vi "Programa_robot_final_5.vi"() -> ()   [LabVIEW 2019]
uses:
  <vilib>/Instr/_visa.llb/VISA Configure Serial Port (Instr).vi
  Global_STOP.vi
  <vilib>/regexp/Match Regular Expression.xnode
panel:
  in  "Ruta hacia el fichero que contiene la imagen de la       superficie del ASIC  fotografiada por el microscopio":path=path "C:/Trabajo_Robot/Test Asic Javi_2021/Origen Socket SERVO_PCB_BUENO_v5 (muchos asics)/capturaQR.jpg"
  in  "stop 6":bool
  in  "Abrir socket 2":bool
  in  "Cerrar socket 2":bool
  in  "Interruptor Error 2":bool
  in  "stop 5":bool
  out "Datos_QR 3":string
  out "Existe foto anterior?":bool
  in  "STOP TEST 3":bool
  in  "stop socket 4":bool
  in  "stop 4":bool
  in  "stop 3":bool
  in  "stop 2":bool
  in  "stop socket 3":bool
  in  "Interruptor Error":bool
  in  "Cerrar socket":bool
  in  "Abrir socket":bool
  out "Error_QR":bool
  out "return count":u32
  out "lectura puerto serie":u32
  out "dato escrito puerto serie":string
  out "OK, Fault 2":bool
  out "error out":errorcluster {"code" format="%f"}
  in  "STOP TEST 2":bool
  out "Datos_QR 2":string
  out "NUMERO ASICS TESTEADOS":i32
  out ".not. x?":bool
  in  "Config File":path=path "C:/Trabajo_Robot/Test Asic Javi_2021/Origen Socket SERVO_PCB_BUENO_v5 (muchos asics)/CONFIG/configuracion_robot_CTAV2022A.test"
  in  "SELECCION DE TEST":string(combo)
  in  "?":bool
  out "Boolean":bool
  in  "stop socket 2":bool
  out "Bytes at port 3":u32=1
  in  "IN y":string(combo)="00"
  in  "IN x":string(combo)="00"
  in  "NOK y":string(combo)="00"
  in  "NOK x":string(combo)="00"
  in  "OK y":string(combo)="00"
  in  "OK x":string(combo)="00"
  in  "Operator's name":string(combo)="Juan Rodríguez"
  in  "?":bool
  in  "Fichero de registro":path=path "C:/Trabajo_Robot/Pruebas/Pruebas.txt"
  in  "Path Out Report":path=path "C:/Trabajo_Robot/desde Marzo 2023/Pruebas_PC_APD/RESULT_TEST_C_LABP0"
  in  "stop socket":bool
  out "Bytes at port 1":u32
  out "Iteraciones":i32
  out "Lectura buffer":string="1"
  in  "Delay (ms)":dbl=1.0 min=1.0 max=9.0 step=1.0
  out "Bytes at port 2":u32=1
  in  "Interruptor":bool=TRUE
  in  "stop":bool
  # "SI SE PRESIONA EL BOTON STOP PARA DETENER EL TEST,\nHAY QUE APAGAR Y VOLVER A ENCENDER EL ARDUINO"
  # "x: columna en cada bandeja \ny: fila en cada bandeja"
  # "Funcionamiento: en la primera iteración, el efector se desplaza desde el origen hasta la celda\nintroducida, hace una pausa, va a la posición del socket (0,0), hace otra pausa, va a la celda\nde salida y vuelve al origen. En las iteraciones siguientes hará lo mismo pero recorriendo las\nceldas de la bandeja sucesivamente. Que el desplazamiento se produzca hacia una celda de\nla bandeja OK o de la bandeja NOK depende de la salidad del programa de test de Asics."
types:
  T1 = enum16{"open", "replace", "create", "open or create", "replace or create", "replace or create with confirmation"}
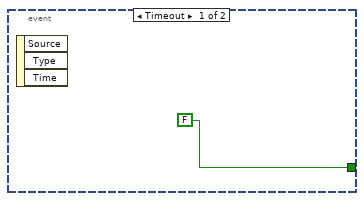
[diagram p2: hidden frame]
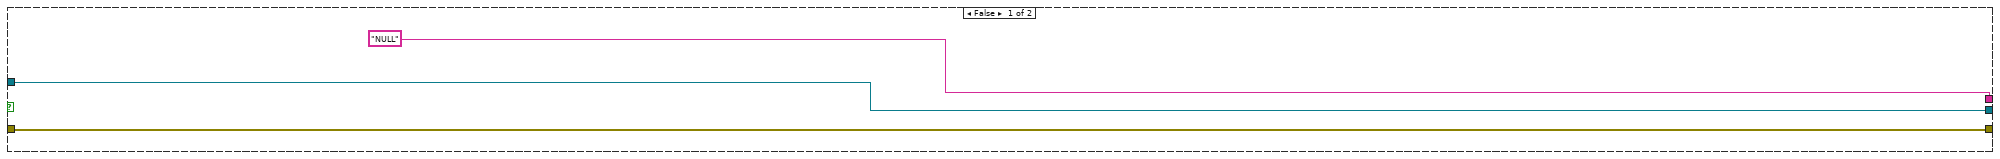
[diagram p5: hidden frame]
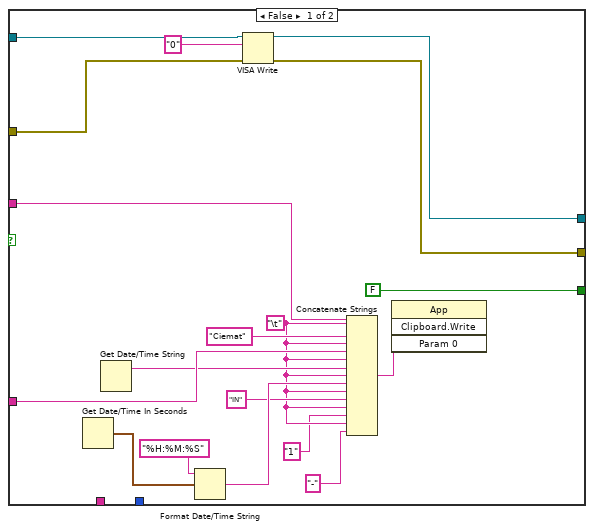
[diagram p8: hidden frame]
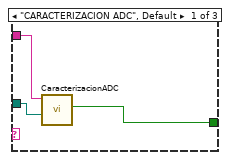
[diagram p9: hidden frame]
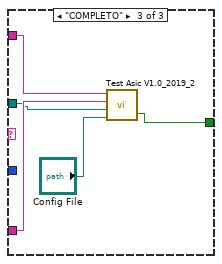
[diagram p10: hidden frame]
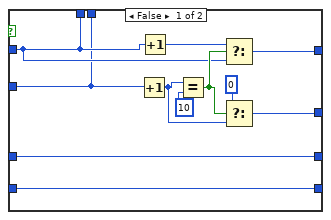
[diagram p12: hidden frame]
diagram:
  n1 = control-ref of="stop socket"() -> (w1:refnum<vi>)
  n2 = control-ref of="Cerrar socket"() -> (w9:refnum<vi>)
  n3 = control-ref of="STOP TEST 2"() -> (w12:refnum<vi>)
  n4 = control-ref of="Abrir socket"() -> (w7:refnum<vi>)
  n5 = control-ref of="stop"() -> (w8:refnum<vi>)
  n6 = control-ref of="Interruptor Error"() -> (w10:refnum<vi>)
  n7 = property class="Bool (strict)"(reference=w12, "Visible"=FALSE) -> ()  [unwired: 1 in, 2 out]
  n8 = property class="Bool (strict)"(reference=w7, "Visible"=FALSE) -> ()  [unwired: 1 in, 2 out]
  n9 = property class="Bool (strict)"(reference=w10, "Visible"=FALSE) -> ()  [unwired: 1 in, 2 out]
  n10 = property class="Bool (strict)"(reference=w9, "Visible"=FALSE) -> ()  [unwired: 1 in, 2 out]
  n11 = property on="Boolean" class="Bool (strict)"("Visible"=FALSE) -> ()  [unwired: 2 in, 2 out]
  n12 = property class="Bool"(reference=w1, "Visible"=FALSE) -> ()  [unwired: 1 in, 2 out]
  n13 = property class="Bool"(reference=w8, "Visible"=FALSE) -> ()  [unwired: 1 in, 2 out]
  n14 = flat-sequence {
    tunnel: [w54] -> w18
    tunnel: ["Fichero de registro"] -> w17
    tunnel: ["SELECCION DE TEST"] -> w16
    tunnel: ["NOK y"] -> w33
    tunnel: ["NOK x"] -> w32
    tunnel: ["OK y"] -> w31
    tunnel: ["OK x"] -> w30
    tunnel: ["IN y"] -> w29
    tunnel: ["IN x"] -> w28
    tunnel: [w57] -> w27
    tunnel: [w58] -> w26
    tunnel: ["IN y"] -> w25
    tunnel: ["IN x"] -> w24
    tunnel: w17 -> [w56]
    frame #0 {
      n15 = while {
        stop <- "?" stop-if-true
        n16 = Not(x="?") -> (.not. x?=w50:bool)
        "Boolean" <- w50
        n17 = property on="Boolean" class="Bool (strict)"("Blinking"=w50) -> ()  [unwired: 2 in, 2 out]
      }
      n18 = global write "Global_STOP.vi" "stop"(FALSE ("stop")) -> ()
    }
    frame #1 {
      n19 = Not(x="?") -> (.not. x?=w54:bool)
      ".not. x?" <- w54
    }
    frame #2 {
      n20 = Open/Create/Replace File(file path (use dialog)=w56, operation (0:open)=T1."open", access (0:read/write)=enum16{"read/write", "read-only", "write-only"}."write-only") -> (refnum out=w69:refnum<file>, error out=w71:errorcluster)  [unwired: 3 in, 1 out]
      n21 = Set File Position(refnum=w69, from (0:start)=enum16{"start", "end", "current"}."end", error in=w71) -> (refnum out=w70:refnum<file>, error out=w72:errorcluster)  [unwired: 1 in]
      n22 = Write to Text File(file (use dialog)=w70, text="\r\n", error in=w72) -> (refnum out=w58:refnum<file>, error out=w57:errorcluster)  [unwired: 1 in, 1 out]
    }
  }
  n23 = Decimal String To Number(string=w25) -> (number=w23:i32)  [unwired: 2 in, 1 out]
  n24 = Decimal String To Number(string=w24) -> (number=w20:i32)  [unwired: 2 in, 1 out]
  n25 = Multiply(x=10, y=w23) -> (x*y=w21:i32)
  n26 = Decimal String To Number(string=w31) -> (number=w35:i32)  [unwired: 2 in, 1 out]
  n27 = Decimal String To Number(string=w30) -> (number=w34:i32)  [unwired: 2 in, 1 out]
  n28 = Decimal String To Number(string=w33) -> (number=w37:i32)  [unwired: 2 in, 1 out]
  n29 = Decimal String To Number(string=w32) -> (number=w36:i32)  [unwired: 2 in, 1 out]
  n30 = call-poly "VISA Configure Serial Port"("VISA resource name"=refnum<visa-resource-name> "COM9", "baud rate (9600)"=u32 9600, "data bits (8)"=u16 8) -> ("VISA resource name out"=w41:refnum<visa-resource-name>, "error out"=w44:errorcluster)  [unwired: 11 in]
  n31 = Add(x=w21, y=w20) -> (x+y=w19:i32)
  n32 = while {
    shift-right: [w82] -> w42
    shift-left: w44 -> [w123]
    tunnel: w41 -> [w121]
    tunnel: [w84] -> w43
    tunnel: w26 -> [w114]
    tunnel: [w113] -> w40
    tunnel: w27 -> [w112]
    tunnel: [w111] -> w39
    tunnel: w28 -> [w109]
    tunnel: w29 -> [w108]
    tunnel: w30 -> [w107]
    tunnel: w31 -> [w106]
    tunnel: w32 -> [w105]
    tunnel: w33 -> [w104]
    shift-right: [w97] -> _
    shift-left: w37 -> [w103]
    shift-right: [w99] -> _
    shift-left: w36 -> [w102]
    shift-right: [w96] -> _
    shift-left: w35 -> [w101]
    shift-right: [w98] -> _
    shift-left: w34 -> [w100]
    tunnel: w19 -> [w95]
    tunnel: w18 -> [w87]
    tunnel: w16 -> [w86]
    tunnel: [w80] -> w14
    i -> [w85]
    stop <- w80 stop-if-true
    n33 = flat-sequence {
      tunnel: w123 -> [w176]
      tunnel: w121 -> [w165]
      tunnel: [w167] -> w120
      tunnel: [w166] -> w119
      tunnel: w109 -> [w146]
      tunnel: w108 -> [w145]
      tunnel: w107 -> [w144]
      tunnel: w106 -> [w143]
      tunnel: w105 -> [w142]
      tunnel: w104 -> [w141]
      tunnel: w120 -> [w913]
      tunnel: w119 -> [w912]
      tunnel: [w911] -> w94
      tunnel: [w910] -> w92
      tunnel: [w909] -> _
      tunnel: w94 -> [w929]
      tunnel: [w927] -> w93
      tunnel: w92 -> [w928]
      tunnel: [w926] -> w91
      tunnel: w93 -> [w949]
      tunnel: w91 -> [w948]
      tunnel: w85 -> [w950]
      tunnel: [w946] -> w90
      tunnel: [w945] -> w89
      tunnel: [w944] -> w88
      tunnel: w85 -> [w1059]
      tunnel: [w1061] -> w117
      tunnel: [w1060] -> w116
      tunnel: [w1057] -> w110
      tunnel: w90 -> [w1056]
      tunnel: w89 -> [w1055]
      tunnel: w88 -> [w1054]
      tunnel: w87 -> [w1049]
      tunnel: w86 -> [w1052]
      tunnel: w85 -> [w1051]
      tunnel: [w1122] -> w115
      tunnel: [w1124] -> w118
      tunnel: w117 -> [w1123]
      tunnel: w116 -> [w1121]
      tunnel: w114 -> [w1128]
      tunnel: [w1127] -> w113
      tunnel: w112 -> [w1126]
      tunnel: [w1125] -> w111
      tunnel: w85 -> [w1118]
      tunnel: w110 -> [w1117]
      tunnel: w103 -> [w1113]
      tunnel: w102 -> [w1116]
      tunnel: w101 -> [w1115]
      tunnel: w100 -> [w1114]
      tunnel: [w1112] -> w97
      tunnel: [w1111] -> w99
      tunnel: [w1110] -> w96
      tunnel: [w1109] -> w98
      tunnel: w95 -> [w1108]
      tunnel: w85 -> [w1107]
      tunnel: [w1106] -> _
      frame #0 {
        n34 = for {
          N: 2 -> [_]
          shift-right: [w788] -> _
          shift-left: w146 -> [w793]
          shift-right: [w791] -> w162
          shift-left: w165 -> [w792]
          shift-right: [w789] -> w161
          shift-left: w176 -> [w790]
          n35 = xnode "Match Regular Expression"("input string"=w793, "regular expression"="-?\\d") -> ("whole match"=w787:string, "after match"=w788:string)  [unwired: 4 in, 3 out]
          n36 = VISA Write(VISA resource name=w792, write buffer=w787, error in (no error)=w790) -> (VISA resource name out=w791:refnum<visa-resource-name>, error out=w789:errorcluster)  [unwired: 1 out]
        }
        n37 = for {
          N: 2 -> [_]
          shift-right: [w666] -> _
          shift-left: w145 -> [w671]
          shift-right: [w669] -> w156
          shift-left: w162 -> [w670]
          shift-right: [w667] -> w155
          shift-left: w161 -> [w668]
          n38 = xnode "Match Regular Expression"("input string"=w671, "regular expression"="-?\\d") -> ("whole match"=w665:string, "after match"=w666:string)  [unwired: 4 in, 3 out]
          n39 = VISA Write(VISA resource name=w670, write buffer=w665, error in (no error)=w668) -> (VISA resource name out=w669:refnum<visa-resource-name>, error out=w667:errorcluster)  [unwired: 1 out]
        }
        n40 = for {
          N: 2 -> [_]
          shift-right: [w544] -> _
          shift-left: w144 -> [w549]
          shift-right: [w547] -> w158
          shift-left: w156 -> [w548]
          shift-right: [w545] -> w157
          shift-left: w155 -> [w546]
          n41 = xnode "Match Regular Expression"("input string"=w549, "regular expression"="-?\\d") -> ("whole match"=w543:string, "after match"=w544:string)  [unwired: 4 in, 3 out]
          n42 = VISA Write(VISA resource name=w548, write buffer=w543, error in (no error)=w546) -> (VISA resource name out=w547:refnum<visa-resource-name>, error out=w545:errorcluster)  [unwired: 1 out]
        }
        n43 = for {
          N: 2 -> [_]
          shift-right: [w422] -> _
          shift-left: w143 -> [w427]
          shift-right: [w425] -> w150
          shift-left: w158 -> [w426]
          shift-right: [w423] -> w149
          shift-left: w157 -> [w424]
          n44 = xnode "Match Regular Expression"("input string"=w427, "regular expression"="-?\\d") -> ("whole match"=w421:string, "after match"=w422:string)  [unwired: 4 in, 3 out]
          n45 = VISA Write(VISA resource name=w426, write buffer=w421, error in (no error)=w424) -> (VISA resource name out=w425:refnum<visa-resource-name>, error out=w423:errorcluster)  [unwired: 1 out]
        }
        n46 = for {
          N: 2 -> [_]
          shift-right: [w300] -> _
          shift-left: w142 -> [w305]
          shift-right: [w303] -> w152
          shift-left: w150 -> [w304]
          shift-right: [w301] -> w151
          shift-left: w149 -> [w302]
          n47 = xnode "Match Regular Expression"("input string"=w305, "regular expression"="-?\\d") -> ("whole match"=w299:string, "after match"=w300:string)  [unwired: 4 in, 3 out]
          n48 = VISA Write(VISA resource name=w304, write buffer=w299, error in (no error)=w302) -> (VISA resource name out=w303:refnum<visa-resource-name>, error out=w301:errorcluster)  [unwired: 1 out]
        }
        n49 = for {
          N: 2 -> [_]
          shift-right: [w178] -> _
          shift-left: w141 -> [w183]
          shift-right: [w181] -> w148
          shift-left: w152 -> [w182]
          shift-right: [w179] -> w147
          shift-left: w151 -> [w180]
          n50 = xnode "Match Regular Expression"("input string"=w183, "regular expression"="-?\\d") -> ("whole match"=w177:string, "after match"=w178:string)  [unwired: 4 in, 3 out]
          n51 = VISA Write(VISA resource name=w182, write buffer=w177, error in (no error)=w180) -> (VISA resource name out=w181:refnum<visa-resource-name>, error out=w179:errorcluster)  [unwired: 1 out]
        }
        n52 = Number To Decimal String(number="Delay (ms)") -> (decimal integer string=w170:string)  [unwired: 1 in]
        n53 = VISA Write(VISA resource name=w148, write buffer=w170, error in (no error)=w147) -> (VISA resource name out=w172:refnum<visa-resource-name>, error out=w171:errorcluster)  [unwired: 1 out]
        n54 = Select(t="1" ("write buffer"), s="Interruptor", f="0" ("write buffer")) -> (s? t:f=w168:string)
        n55 = VISA Write(VISA resource name=w172, write buffer=w168, error in (no error)=w171) -> (VISA resource name out=w167:refnum<visa-resource-name>, error out=w166:errorcluster)  [unwired: 1 out]
      }
      frame #1 {
        n56 = while {
          shift-right: [w919] -> w910
          shift-left: w912 -> [w924]
          tunnel: ["stop socket"] -> _
          shift-right: [w920] -> w911
          shift-left: w913 -> [w925]
          tunnel: ["stop socket"] -> w909
          stop <- w914 stop-if-true
          n57 = property class="Instr"(reference=w925, error in=w924) -> (reference out=w923:refnum<visa-resource-name>, error out=w922:errorcluster, "Bytes at Port"=w921:u32)
          "Bytes at port 1" <- w921
          n58 = VISA Read(VISA resource name=w923, byte count=w921, error in (no error)=w922) -> (VISA resource name out=w920:refnum<visa-resource-name>, read buffer=w918:string, error out=w919:errorcluster)  [unwired: 1 out]
          n59 = Equal?(x="2", y=w918) -> (x = y?=w916:bool)
          n60 = Or(x=w916, y="stop socket") -> (x .or. y?=w914:bool)
        }
      }
      frame #2 {
        n61 = while {
          shift-right: [w935] -> w926
          shift-left: w928 -> [w940]
          tunnel: ["stop socket 2"] -> _
          shift-right: [w936] -> w927
          shift-left: w929 -> [w941]
          tunnel: ["stop socket 2"] -> _
          stop <- w930 stop-if-true
          n62 = property class="Instr"(reference=w941, error in=w940) -> (reference out=w939:refnum<visa-resource-name>, error out=w938:errorcluster, "Bytes at Port"=w937:u32)
          "Bytes at port 3" <- w937
          n63 = VISA Read(VISA resource name=w939, byte count=w937, error in (no error)=w938) -> (VISA resource name out=w936:refnum<visa-resource-name>, read buffer=w934:string, error out=w935:errorcluster)  [unwired: 1 out]
          n64 = Equal?(x="3", y=w934) -> (x = y?=w932:bool)
          n65 = Or(x=w932, y="stop socket 2") -> (x .or. y?=w930:bool)
        }
      }
      frame #3 {
        # "Este bloque realiza la captura y lectura del QR"
        n66 = Greater?(x=w950, y=-1) -> (0:w947:bool)
        n67 = case shown="True" w947 {
          tunnel: [w954 w956] -> w944
          tunnel: w949 -> [w954 w958]
          tunnel: [w953 w957] -> w946
          tunnel: w948 -> [w953 w959]
          tunnel: ["NULL" ("Datos_QR") w955] -> w945
          frame False {
          }
          frame True {
            n68 = while {
              tunnel: [w965] -> w955
              tunnel: w958 -> [w976]
              tunnel: [w972] -> w956
              tunnel: [w971] -> w957
              tunnel: w959 -> [w966]
              stop <- w961 stop-if-true
              n69 = flat-sequence {
                tunnel: [w980] -> w967
                tunnel: w966 -> [w978]
                tunnel: [w992] -> w965
                tunnel: [w990] -> w962
                tunnel: w967 -> [w989]
                tunnel: [w989] -> w964
                frame #0 {
                  # "Éste bloque borra el fichero de imagen\ndel Asic anterior."
                  n70 = call <vilib>:"Check if File or Folder Exists.vi"("error in (no error)"=w978, "path"="Ruta hacia el fichero que contiene la imagen de la       superficie del ASIC  fotografiada por el microscopio") -> ("error out"=w979:errorcluster, "file or folder exists?"=w982:bool, "dup path"=w981:path)  [unwired: 7 in]
                  "Existe foto anterior?" <- w982
                  n71 = case shown="True" w982 {
                    tunnel: w981 -> [w984 w988]
                    tunnel: [w984 w987] -> _
                    tunnel: [w983 w986] -> w980
                    tunnel: w979 -> [w983 w985]
                    frame False {
                    }
                    frame True {
                      n72 = Delete(path (use dialog)=w988, error in=w985) -> (deleted path=w987:path, error out=w986:errorcluster)  [unwired: 3 in, 1 out]
                    }
                  }
                }
                frame #1 {
                  # "Éste bloque realiza la captura de imagen\ndel QR del asic para leer el código."
                  n73 = for {
                    N: 5 -> [_]
                    tunnel: [w997] -> w992
                    tunnel: [w995] -> w990
                    stop <- w993 stop-if-true
                    n74 = call "CapturaImagenyQR_subVI.vi"() -> ("Datos_QR"=w997:string)  [unwired: 11 in]
                    "Datos_QR 3" <- w997
                    n75 = Equal?(x=w997, y="" ("Datos_QR")) -> (x = y?=w996:bool)
                    n76 = global read "Global_STOP.vi" "stop"() -> (w994:bool)
                    n77 = Not(x=w996) -> (.not. x?=w995:bool)
                    n78 = Compound Arithmetic op=OR(w995, w994) -> (w993:bool)
                  }
                }
              }
              n79 = Select(t="1" ("write buffer"), s=w962, f="0" ("write buffer")) -> (s? t:f=w973:string)
              n80 = Not(x=w962) -> (.not. x?=→"Error_QR":bool)
              n81 = VISA Write(VISA resource name=w976, write buffer=w973, error in (no error)=w964) -> (VISA resource name out=w970:refnum<visa-resource-name>, error out=w969:errorcluster)  [unwired: 1 out]
              n82 = global read "Global_STOP.vi" "stop"() -> (w963:bool)
              n83 = case shown="False" w962 {
                tunnel: w970 -> [w1010 w1045]
                tunnel: w969 -> [w1009 w1044]
                tunnel: [w1008 w1045] -> w972
                tunnel: [w1007 w1044] -> w971
                frame False {
                  n84 = flat-sequence {
                    tunnel: w1010 -> [w1014]
                    tunnel: [w1013] -> w1006
                    tunnel: [w1012] -> w1004
                    tunnel: w1009 -> [w1011]
                    tunnel: w1006 -> [w1025]
                    tunnel: [w1025] -> w1005
                    tunnel: w1004 -> [w1024]
                    tunnel: [w1024] -> w1003
                    tunnel: w1005 -> [w1029]
                    tunnel: w1003 -> [w1028]
                    tunnel: [w1027] -> w1002
                    tunnel: [w1026] -> w1000
                    tunnel: w1002 -> [w1040]
                    tunnel: [w1040] -> w1001
                    tunnel: w1000 -> [w1039]
                    tunnel: [w1039] -> w999
                    tunnel: [w1041] -> w1007
                    tunnel: [w1042] -> w1008
                    tunnel: w1001 -> [w1042]
                    tunnel: w999 -> [w1041]
                    frame #0 {
                      n85 = while {
                        tunnel: w1014 -> [w1022]
                        tunnel: [w1017] -> w1013
                        tunnel: [w1016] -> w1012
                        tunnel: w1011 -> [w1015]
                        stop <- "Abrir socket" stop-if-true
                        n86 = Select(t="2" ("write buffer"), s="Abrir socket", f="0" ("write buffer")) -> (s? t:f=w1019:string)
                        n87 = VISA Write(VISA resource name=w1022, write buffer=w1019, error in (no error)=w1015) -> (VISA resource name out=w1017:refnum<visa-resource-name>, error out=w1016:errorcluster)  [unwired: 1 out]
                      }
                    }
                    frame #1 {
                      n88 = Wait (ms)(milliseconds to wait=u32 1000) -> ()  [unwired: 1 out]
                    }
                    frame #2 {
                      n89 = while {
                        tunnel: w1029 -> [w1033]
                        tunnel: w1028 -> [w1032]
                        tunnel: [w1031] -> w1027
                        tunnel: [w1030] -> w1026
                        stop <- "Cerrar socket" stop-if-true
                        n90 = Select(t="3" ("write buffer"), s="Cerrar socket", f="0" ("write buffer")) -> (s? t:f=w1035:string)
                        n91 = VISA Write(VISA resource name=w1033, write buffer=w1035, error in (no error)=w1032) -> (VISA resource name out=w1031:refnum<visa-resource-name>, error out=w1030:errorcluster)  [unwired: 1 out]
                      }
                    }
                    frame #3 {
                      n92 = Wait (ms)(milliseconds to wait=u32 1000) -> ()  [unwired: 1 out]
                    }
                    frame #4 {
                      n93 = while {
                        stop <- "Interruptor Error" stop-if-true
                      }
                    }
                  }
                }
                frame True {
                }
              }
              n94 = Or(x=w962, y=w963) -> (x .or. y?=w961:bool)
            }
            n95 = Wait (ms)(milliseconds to wait=u32 10000) -> ()  [unwired: 1 out]
          }
        }
        n96 = control-ref of="STOP TEST 2"() -> (w943:refnum<vi>)
        n97 = property class="Bool (strict)"(reference=w943, "Visible"=TRUE) -> ()  [unwired: 1 in, 2 out]
      }
      frame #4 {
        n98 = global read "Global_STOP.vi" "stop"() -> (w1048:bool)
        n99 = Greater?(x=w1059, y=-1) -> (0:w1050:bool)
        n100 = Not(x=w1048) -> (.not. x?=w1047:bool)
        n101 = Compound Arithmetic op=AND(w1050, w1049, w1047) -> (w1046:bool)
        n102 = case shown="True" w1046 {
          tunnel: w1054 -> [w1077 w1084]
          tunnel: w1056 -> [w1076 w1083]
          tunnel: [w1075 w1082] -> w1061
          tunnel: [w1074 w1081] -> w1060
          tunnel: w1055 -> [w1070 w1091]
          tunnel: [FALSE ("Boolean") w1089] -> w1057
          tunnel: "Operator's name" -> [w1068 w1088]
          tunnel: w1052 -> [_ w1087]
          tunnel: w1051 -> [_ w1086]
          frame False {
            w1064 = "\t"
            n103 = Get Date/Time In Seconds() -> (seconds since 1Jan1904=w1072:timestamp)
            n104 = Get Date/Time String() -> (date string=w1067:string)  [unwired: 3 in, 1 out]
            n105 = Format Date/Time String(time format string (%c)="%H:%M:%S", seconds (now)=w1072) -> (date/time string=w1066:string)  [unwired: 1 in]
            n106 = VISA Write(VISA resource name=w1077, write buffer="0", error in (no error)=w1076) -> (VISA resource name out=w1075:refnum<visa-resource-name>, error out=w1074:errorcluster)  [unwired: 1 out]
            n107 = Concatenate Strings(w1070, w1064, "Ciemat", w1064, w1068, w1064, w1067, w1064, w1066, w1064, "IN", w1064, "1", w1064, "-") -> (w1073:string)
            n108 = invoke class="App" method="Clipboard.Write"("Param 0"=w1073) -> ()  [unwired: 3 in, 4 out]
          }
          frame True {
            # "Test de Asics"
            n109 = case shown="\"SUMAS 3 CANALES\"" w1087 {
              tunnel: w1091 -> [w1096 w1098 w1105]
              tunnel: "Path Out Report" -> [w1095 w1100 w1103]
              tunnel: [w1094 w1099 w1101] -> w1089
              tunnel: w1088 -> [_ _ w1104]
              tunnel: w1086 -> [_ w1097 _]
              frame "CARACTERIZACION ADC", Default {
                n110 = call "CaracterizacionADC.vi"("QR code"=w1096, "Path Out Report"=w1095) -> ("OK/NOK"=w1094:bool)  [unwired: 7 in]
              }
              frame "SUMAS 3 CANALES" {
                n111 = call "Test_Sumadores_Javi.vi"("QR"=w1098, "Path"=w1100, "NUMERO DE PASADA DE TEST"=w1097) -> ("Boolean"=w1099:bool)  [unwired: 8 in]
                "NUMERO ASICS TESTEADOS" <- w1097
              }
              frame "COMPLETO" {
                n112 = call "Test Asic V1.0_2019_2.vi"("Config File"="Config File", "Path Out Report"=w1103, "Operator's Name"=w1104, "ASIC'S Number"=w1105) -> ("OK, Fault 2"=w1101:bool)  [unwired: 1 in]
              }
            }
            "OK, Fault 2" <- w1089
            n113 = Select(t="1" ("write buffer"), s=w1089, f="0" ("write buffer")) -> (s? t:f=w1085:string)
            "dato escrito puerto serie" <- w1085
            n114 = VISA Write(VISA resource name=w1084, write buffer=w1085, error in (no error)=w1083) -> (VISA resource name out=w1082:refnum<visa-resource-name>, return count=→"return count":u32, error out=w1081:errorcluster)
          }
        }
      }
      frame #5 {
        n115 = Greater?(x=w1118, y=-1) -> (0:w1119:bool)
        n116 = case shown="True" w1119 {
          tunnel: w1128 -> [w1134 w1167]
          tunnel: [w1134 w1166] -> w1127
          tunnel: w1126 -> [w1133 w1165]
          tunnel: [w1133 w1164] -> w1125
          tunnel: [w1136 w1163] -> w1124
          tunnel: w1123 -> [w1136 w1163]
          tunnel: [w1135 w1162] -> w1122
          tunnel: w1121 -> [w1135 w1162]
          tunnel: w1117 -> [_ w1160]
          tunnel: w1113 -> [w1132 w1159]
          tunnel: w1116 -> [w1131 w1158]
          tunnel: w1115 -> [w1130 w1157]
          tunnel: w1114 -> [w1129 w1156]
          tunnel: [w1132 w1155] -> w1112
          tunnel: [w1131 w1154] -> w1111
          tunnel: [w1130 w1153] -> w1110
          tunnel: [w1129 w1152] -> w1109
          frame False {
          }
          frame True {
            w1139 = "\t"
            # "Registro de datos en fichero"
            n117 = invoke class="App" method="Clipboard.Read"() -> ("Read Clipbrd"=w1161:string)  [unwired: 3 in, 2 out]
            n118 = case shown="True" w1160 {
              tunnel: w1159 -> [w1170 w1183]
              tunnel: w1158 -> [w1169 w1182]
              tunnel: w1157 -> [w1172 w1180]
              tunnel: w1156 -> [w1171 w1181]
              tunnel: [w1174 w1183] -> w1155
              tunnel: [w1173 w1182] -> w1154
              tunnel: [w1172 w1185] -> w1153
              tunnel: [w1171 w1184] -> w1152
              tunnel: [w1170 w1180] -> w1151
              tunnel: [w1169 w1181] -> w1150
              frame False {
                n119 = Increment(x=w1169) -> (x+1=w1178:i32)
                n120 = Increment(x=w1170) -> (x+1=w1175:i32)
                n121 = Equal?(x=w1178, y=10) -> (x = y?=w1176:bool)
                n122 = Select(t=w1175, s=w1176, f=w1170) -> (s? t:f=w1174:i32)
                n123 = Select(t=0, s=w1176, f=w1178) -> (s? t:f=w1173:i32)
              }
              frame True {
                n124 = Increment(x=w1181) -> (x+1=w1189:i32)
                n125 = Increment(x=w1180) -> (x+1=w1186:i32)
                n126 = Equal?(x=w1189, y=10) -> (x = y?=w1187:bool)
                n127 = Select(t=w1186, s=w1187, f=w1180) -> (s? t:f=w1185:i32)
                n128 = Select(t=0, s=w1187, f=w1189) -> (s? t:f=w1184:i32)
              }
            }
            n129 = Write to Text File(file (use dialog)=w1167, text=w1161, error in=w1165) -> (refnum out=w1148:refnum<file>, error out=w1149:errorcluster)  [unwired: 1 in, 1 out]
            n130 = Number To Decimal String(number=w1151) -> (decimal integer string=w1138:string)  [unwired: 1 in]
            n131 = Number To Decimal String(number=w1150) -> (decimal integer string=w1137:string)  [unwired: 1 in]
            n132 = Write to Text File(file (use dialog)=w1148, text=w1139, error in=w1149) -> (refnum out=w1146:refnum<file>, error out=w1147:errorcluster)  [unwired: 1 in, 1 out]
            n133 = Write to Text File(file (use dialog)=w1146, text=w1138, error in=w1147) -> (refnum out=w1143:refnum<file>, error out=w1142:errorcluster)  [unwired: 1 in, 1 out]
            n134 = Write to Text File(file (use dialog)=w1143, text=w1139, error in=w1142) -> (refnum out=w1141:refnum<file>, error out=w1140:errorcluster)  [unwired: 1 in, 1 out]
            n135 = Write to Text File(file (use dialog)=w1141, text=w1137, error in=w1140) -> (refnum out=w1145:refnum<file>, error out=w1144:errorcluster)  [unwired: 1 in, 1 out]
            n136 = Write to Text File(file (use dialog)=w1145, text="\r\n", error in=w1144) -> (refnum out=w1166:refnum<file>, error out=w1164:errorcluster)  [unwired: 1 in, 1 out]
          }
        }
        n137 = Add(x=w1108, y=w1107) -> (x+y=w1106:i32)
      }
    }
    n138 = while {
      shift-right: [w1198] -> w76
      shift-left: w115 -> [w1204]
      tunnel: ["stop"] -> _
      shift-right: [w1199] -> w84
      shift-left: w118 -> [w1205]
      tunnel: [w1194] -> w122
      stop <- w1192 stop-if-true
      # "1"
      # "Mientras se ejecuta este bucle (la espera a que\nArduino termine una iteración), cambiamos los\ndatos de los controladores."
      n139 = property class="Instr"(reference=w1205, error in=w1204) -> (reference out=w1202:refnum<visa-resource-name>, error out=w1201:errorcluster, "Bytes at Port"=w1200:u32)
      "Bytes at port 2" <- w1200
      n140 = VISA Read(VISA resource name=w1202, byte count=w1200, error in (no error)=w1201) -> (VISA resource name out=w1199:refnum<visa-resource-name>, read buffer=w1194:string, return count=w1197:u32, error out=w1198:errorcluster)
      "lectura puerto serie" <- w1197
      n141 = Greater Or Equal?(x=w1197, y=u32 1) -> (x >= y?=w1195:bool)
      n142 = global read "Global_STOP.vi" "stop"() -> (w1191:bool)
      n143 = Or(x=w1195, y="stop") -> (x .or. y?=w1193:bool)
      n144 = Compound Arithmetic op=OR(w1193, w1191) -> (w1192:bool)
    }
    "Lectura buffer" <- w122
    n145 = flat-sequence {
      tunnel: w76 -> [w125]
      tunnel: [w125] -> w75
      tunnel: [w124] -> w73
      frame #0 {
        n146 = global read "Global_STOP.vi" "stop"() -> (w124:bool)
      }
    }
    n147 = case shown="False" w73 {
      selector: w73 -> [_ w135]
      tunnel: [w129 _] -> w81
      tunnel: [w126 w135] -> w77
      tunnel: w75 -> [w127 w134]
      tunnel: [w127 w134] -> w74
      frame False {
        n148 = for {
          N: 3 -> [_]
          tunnel: [w132] -> _
          tunnel: [w130] -> w129
          tunnel: [w130] -> w126
          stop <- w130 stop-if-true
          n149 = call "CapturaImagenyQR_subVI.vi"() -> ("Datos_QR"=w132:string)  [unwired: 11 in]
          "Datos_QR 2" <- w132
          n150 = Equal?(x=w132, y="" ("Datos_QR")) -> (x = y?=w131:bool)
          n151 = Not(x=w131) -> (.not. x?=w130:bool)
        }
      }
      frame True {
      }
    }
    n152 = flat-sequence {
      tunnel: [w138] -> w80
      tunnel: w77 -> [w136]
      frame #0 {
        n153 = global read "Global_STOP.vi" "stop"() -> (w137:bool)
        n154 = Or(x=w136, y=w137) -> (x .or. y?=w138:bool)
      }
    }
    n155 = Boolean To (0,1)(Boolean=w81) -> (0, 1=w79:i16)
    n156 = call <vilib>:"Error Cluster From Error Code.vi"("error in (no error)"=w74, "error message (\"\")"="El asic no se ha colocado en la\n    bandeja de salida,se ha quedado\nen el socket posiblemente por una\nmala succión de la ventosa.\nPresione STOP\n" ("error message (\"\")"), "error code (0)"=w79) -> ("error out"=w78:errorcluster)  [unwired: 6 in]
    n157 = call <vilib>:"Simple Error Handler.vi"("error in (no error)"=w78) -> ("error out"=w82:errorcluster)  [unwired: 4 in, 4 out]
    n158 = case shown="True" w81 {
      selector: w81 -> [w139 w140]
      tunnel: [w139 w140] -> _
      frame False {
      }
      frame True {
        n159 = call "Send Email2"() -> ()  [unwired: 11 in, 1 out]
      }
    }
    "Iteraciones" <- w85
  }
  n160 = flat-sequence {
    frame #0 {
      n161 = local write "STOP TEST 2"(FALSE ("STOP TEST 2")) -> ()
    }
    frame #1 {
      n162 = while {
        stop <- w1207 stop-if-true
        n163 = event shown="[1] \"STOP TEST 2\": Value Change" {
          selector: _ -> [_ _]
          dyn-events: _ -> [_ _]
          timeout: _ -> [_ _]
          tunnel: [FALSE "STOP TEST 2"] -> w1207
          event Timeout {
            n164 = event-data() -> ()  [unwired: 1 in, 3 out]
          }
          event "STOP TEST 2": Value Change {
            n165 = event-data() -> ()  [unwired: 1 in, 6 out]
            n166 = global write "Global_STOP.vi" "stop"("STOP TEST 2") -> ()
            n167 = Wait (ms)(milliseconds to wait=u32 100) -> ()  [unwired: 1 out]
          }
        }
      }
    }
  }
  n168 = Close File(refnum=w40, error in=w39) -> (error out=w38:errorcluster)  [unwired: 1 out]
  n169 = Not(x=w14) -> (.not. x?=w15:bool)
  n170 = call <vilib>:"Simple Error Handler.vi"("error in (no error)"=w38) -> ()  [unwired: 4 in, 5 out]
  n171 = global write "Global_STOP.vi" "stop"(w15) -> ()
  n172 = VISA Close(VISA resource name=w43, error in (no error)=w42) -> (error out=→"error out":errorcluster)
